vi "Run.vi"(8 "error in (no error)":errorcluster, 11 "Car Wash Console in":refnum<class "Car Wash Console.lvclass">) -> (0 "error out":errorcluster, 3 "Car Wash Console out":refnum<class "Car Wash Console.lvclass">)   [LabVIEW 2016, in "CLD Exam - Car Wash.lvlib" / "Car Wash Console.lvclass"]
doc: "--\nCopyright © 2017 Composed SystemsI All rights reserved.\n\nAuthor: Jon McBee <jon.mcbee@composed.io>\n\nThis library is provided \"AS IS\" ,WITHOUT WARRANTIES OR\nCONDITIONS OF ANY KIND, either express or implied.\n\nComposed Systems -- composed.io\n\nStream 0.0.1.1\nJon McBee - Composed Systems\nCopyright (c) 2017, Composed Systems"
uses:
  Car Wash Console.lvclass
  D:/Repos/Stream/software/Mediator/Classes/Mediated Actor/Mediated Actor.lvclass
  Mediator/Classes/Message Interface/Message Interface.lvclass
  Car Wash Console.lvclass/Car Wash Console.ctl
  Car Wash Started Event/Car Wash Started.lvclass
  D:/Repos/Stream/software/Mediator/Classes/Message Interface/Message Interface.lvclass
  Mediator/Classes/Message Transport Queue/Message Transport Queue.lvclass
  Mediator/Classes/Mediated Actor/Mediated Actor.lvclass
panel:
  out "Alpha":bool
  in  "Start":bool
  in  "Air Dry":bool
  in  "Tire Shine Foam":bool
  in  "Spot Free Rinse":bool
  in  "Low Pressure Wax":bool
  in  "High Pressure Wash":bool
  in  "Pre-Soak":bool
  in  "Bug Remover":bool
  in  "Under Body Wash":bool
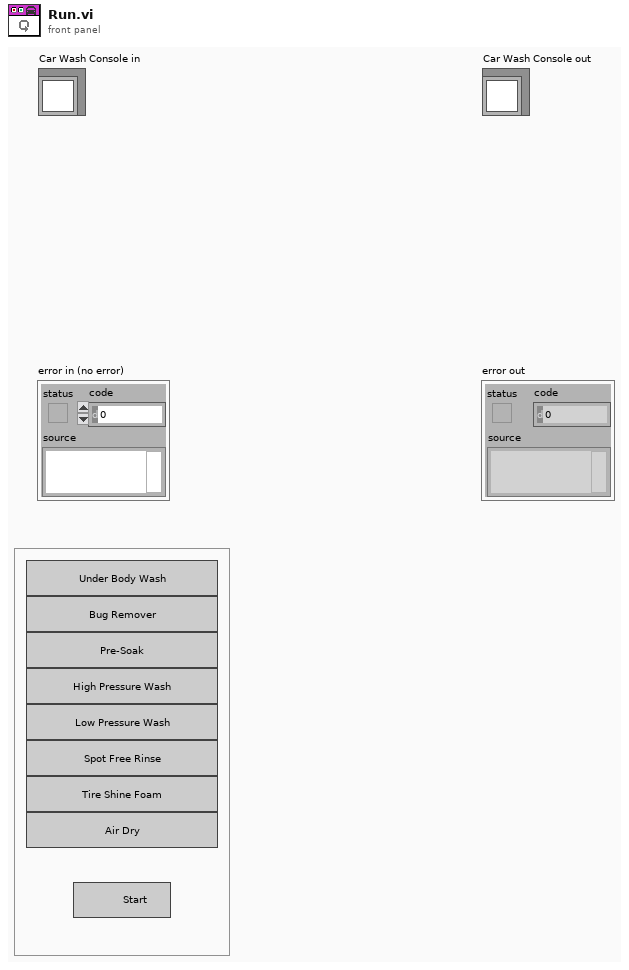
[diagram p1: front panel]
types:
  T1 = cluster{"System Exit":refnum<event-registration>, "To Self":refnum<event-registration>, "Car Wash Finished":refnum<event-registration>}
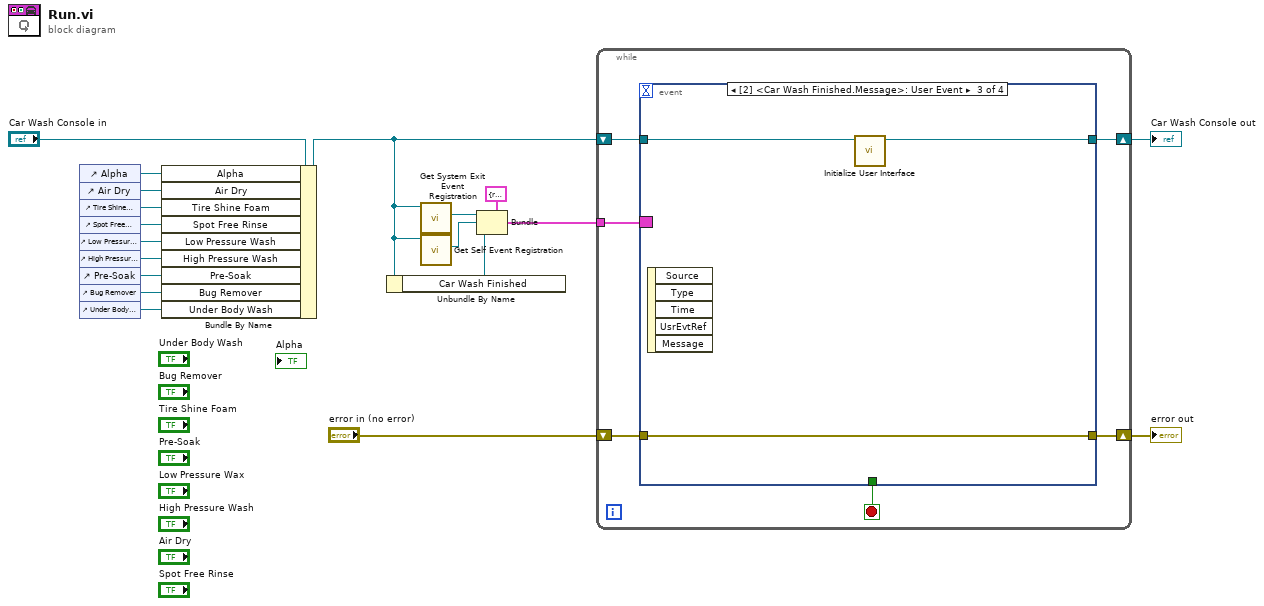
[diagram p0: block diagram]
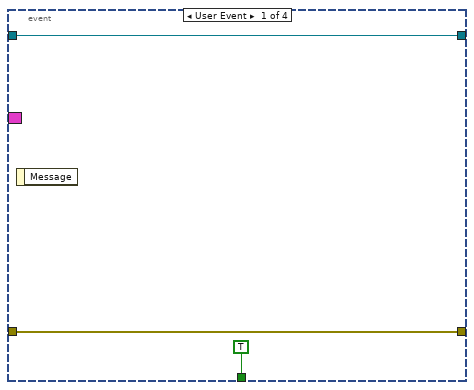
[diagram p2: hidden frame]
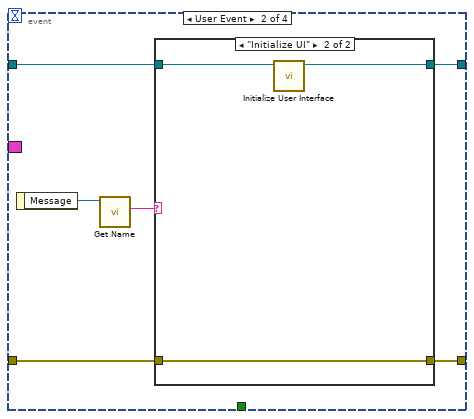
[diagram p3: hidden frame]
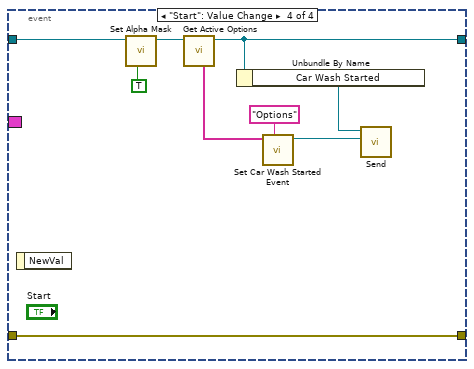
[diagram p5: hidden frame]
diagram:
  n1 = control-ref of="Alpha"() -> (w12:refnum<vi>)
  n2 = control-ref of="Air Dry"() -> (w11:refnum<vi>)
  n3 = control-ref of="Tire Shine Foam"() -> (w10:refnum<vi>)
  n4 = control-ref of="Spot Free Rinse"() -> (w9:refnum<vi>)
  n5 = control-ref of="Low Pressure Wax"() -> (w8:refnum<vi>)
  n6 = control-ref of="High Pressure Wash"() -> (w7:refnum<vi>)
  n7 = control-ref of="Pre-Soak"() -> (w6:refnum<vi>)
  n8 = control-ref of="Bug Remover"() -> (w5:refnum<vi>)
  n9 = control-ref of="Under Body Wash"() -> (w4:refnum<vi>)
  n10 = Bundle By Name(cluster="Car Wash Console in", "Alpha"=w12, "Air Dry"=w11, "Tire Shine Foam"=w10, "Spot Free Rinse"=w9, "Low Pressure Wash"=w8, "High Pressure Wash"=w7, "Pre-Soak"=w6, "Bug Remover"=w5, "Under Body Wash"=w4) -> (w3:refnum<class "Car Wash Console.lvclass">)
  n11 = Unbundle By Name(w3) -> ("Car Wash Finished"=w1:refnum<event-registration>)
  n12 = call "Get System Exit Event Registration.vi"("Mediated Actor in"=w3) -> ("System Exit Registration"=w16:refnum<event-registration>)  [unwired: 9 in, 1 out]
  n13 = call "Get Self Event Registration.vi"("Mediated Actor in"=w3) -> ("Event Registration Refnum"=w15:refnum<event-registration>)  [unwired: 9 in, 1 out]
  n14 = Bundle(cluster=T1 {"System Exit"=refnum, "To Self"=refnum, "Car Wash Finished"=refnum} ("output cluster"), "System Exit"=w16, "To Self"=w15, "Car Wash Finished"=w1) -> (w14:T1)
  n15 = while {
    shift-right: [w24] -> w18
    shift-left: "error in (no error)" -> [w25]
    shift-right: [w22] -> w17
    shift-left: w3 -> [w23]
    tunnel: w14 -> [w21]
    stop <- w20 stop-if-true
    n16 = event shown="[2] <Car Wash Finished.Message>: User Event" {
      selector: w21 -> [_ _ _ _]
      dyn-events: _ -> [_ _ _ _]
      timeout: _ -> [_ _ _ _]
      tunnel: w25 -> [w28 w30 w42 w51]
      tunnel: [w28 w29 w42 w51] -> w24
      tunnel: w23 -> [w27 w32 w41 w49]
      tunnel: [w27 w31 w40 w44] -> w22
      tunnel: [TRUE _ _ _] -> w20
      event User Event {
        n17 = event-data() -> ()  [unwired: 1 in, 1 out]
      }
      event User Event {
        n18 = event-data() -> ("Message"=w34:refnum<class "Message Interface.lvclass">)  [unwired: 1 in]
        n19 = call "Get Name.vi"("Message Interface in"=w34) -> ("Name"=w33:string)  [unwired: 8 in, 2 out]
        n20 = case shown="\"Initialize UI\"" w33 {
          tunnel: [w36 w37] -> w31
          tunnel: w32 -> [w36 w38]
          tunnel: [w35 w39] -> w29
          tunnel: w30 -> [w35 w39]
          frame Default {
          }
          frame "Initialize UI" {
            n21 = call "Initialize User Interface.vi"("Car Wash Console in"=w38) -> ("Car Wash Console out"=w37:refnum<class "Car Wash Console.lvclass">)  [unwired: 9 in, 1 out]
          }
        }
      }
      event User Event {
        n22 = event-data() -> ()  [unwired: 1 in, 5 out]
        n23 = call "Initialize User Interface.vi"("Car Wash Console in"=w41) -> ("Car Wash Console out"=w40:refnum<class "Car Wash Console.lvclass">)  [unwired: 9 in, 1 out]
      }
      event "Start": Value Change {
        n24 = event-data() -> ()  [unwired: 1 in, 1 out]
        n25 = call "Set Alpha Mask.vi"("Mask?"=TRUE ("Visible"), "Car Wash Console in"=w49) -> ("Car Wash Console out"=w47:refnum<class "Car Wash Console.lvclass">)  [unwired: 8 in, 1 out]
        n26 = call "Get Active Options.vi"("Car Wash Console in"=w47) -> ("Car Wash Console out"=w44:refnum<class "Car Wash Console.lvclass">, "Options"=w46:string[])  [unwired: 9 in]
        n27 = Unbundle By Name(w44) -> ("Car Wash Started"=w43:refnum<class "Message Transport Queue.lvclass">)
        n28 = call "Set Car Wash Started Event.vi"("Name"="Options", "Wash Options"=w46) -> ("Car Wash Started out"=w50:refnum<class "Car Wash Started.lvclass">)  [unwired: 8 in, 1 out]
        n29 = call-dynamic "Send.vi"("Message"=w50, "Message Transport Queue in"=w43) -> ()  [unwired: 7 in, 3 out]
      }
    }
  }
  "error out" <- w18
  "Car Wash Console out" <- w17
